vi "Init.vi"(8 "error in (no error)":errorcluster) -> (0 "error out":errorcluster, 3 "Message Queues out":T1)   [LabVIEW 2017, in "Server.lvlib"]
doc: "This VI creates all Message Queues and User Events, initializes the ErrorHandler and the Stop-Global Variable."
uses:
  Server.lvlib
  SubLibs/Message Queue/CommReferences.ctl
  SubLibs/Message Queue/MessageCluster.ctl
  SubLibs/Message Queue/EnqueueMessage(Single).vi
  SubLibs/Message Queue/Message Queue.lvlib
  SubLibs/ErrorLogger/ErrorLogger.lvlib
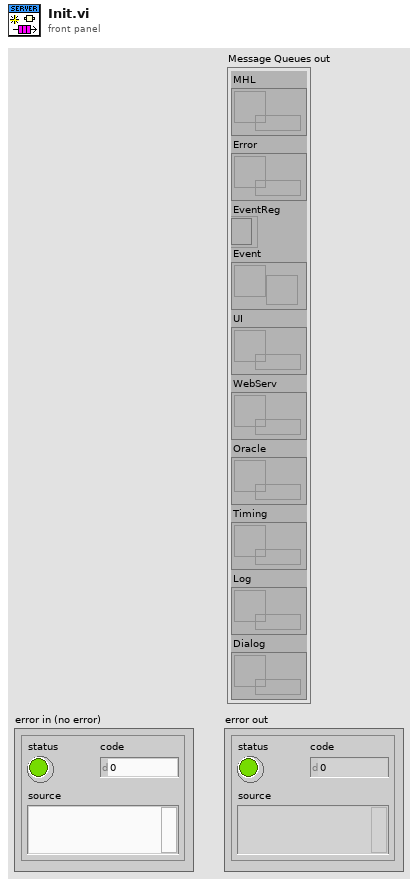
[diagram p1: front panel]
types:
  T1 = typedef "Server.lvlib/Message Queue.lvlib/CommReferences.ctl" = cluster{"MHL":refnum<queue>, "Error":refnum<queue>, "EventReg":refnum<event-registration>, "Event":refnum<user-event>, "UI":refnum<queue>, "WebServ":refnum<queue>, "Oracle":refnum<queue>, "Timing":refnum<queue>, "Log":refnum<queue>, "Dialog":refnum<queue>}
  T2 = typedef "Server.lvlib/ServerINI.ctl" = cluster{"ClientTimeout (s)":u32, "LogPath":path, "CriticalErrors":i32[], "OracleData":T3}
  T3 = typedef "Server.lvlib/Oracle.lvlib/OracleData.ctl" = cluster{"DBname":string, "User":string, "Password":string}
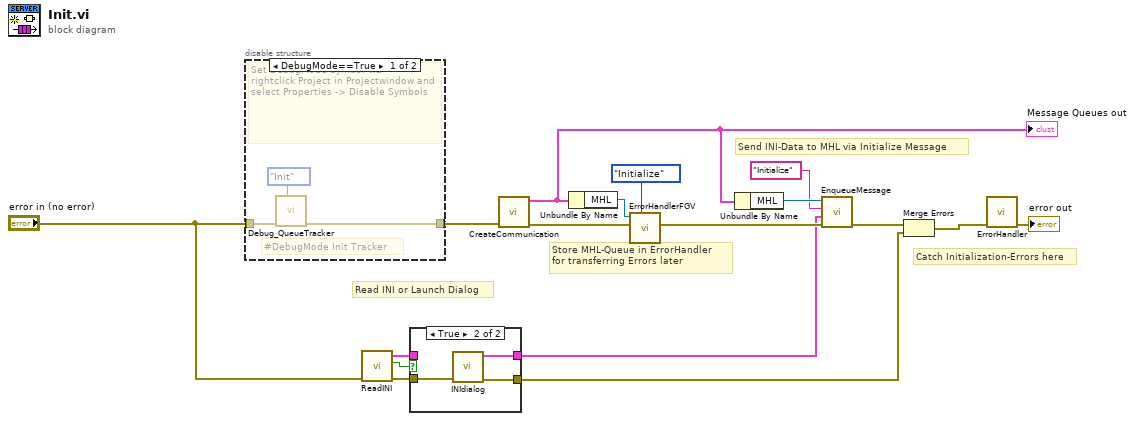
[diagram p0: block diagram]
diagram:
  # "Catch Initialization-Errors here"
  # "Send INI-Data to MHL via Initialize Message"
  # "Store MHL-Queue in ErrorHandler\nfor transferring Errors later"
  # "Read INI or Launch Dialog"
  n1 = disable-structure shown="DebugMode==True" {
    disable-tunnel: "error in (no error)" -> [w19 w21]
    disable-tunnel: [w18 w21] -> w10
    frame condition #0 {
      # "#DebugMode Init Tracker"
      # "Set DebugMode-Symbol via\nrightclick Project in Projectwindow and select Properties -> Disable Symbols"
      n2 = call "Debug_QueueTracker.vi"("Mode"=enum16{"Init", "Track", "DeInit"}."Init", "Error In"=w19) -> ("Error Out"=w18:errorcluster)  [unwired: 9 in]
    }
    frame condition #1 (active) {
      # "Don't track Queues if not in \nDebug-Mode.\nMode is settable in Project-file"
    }
  }
  n3 = call "ReadINI.vi"("error in (no error)"="error in (no error)") -> ("error out"=w12:errorcluster, "FileNotFound/Corrupted?"=w11:bool, "value"=w9:T2)  [unwired: 8 in]
  n4 = case shown="True" w11 {
    tunnel: w12 -> [w23 w26]
    tunnel: [w23 w25] -> w1
    tunnel: [w22 w24] -> w4
    tunnel: w9 -> [w22 _]
    frame False {
    }
    frame True {
      n5 = call "INIdialog.vi"("Error In"=w26) -> ("Error Out"=w25:errorcluster, "ServerINI"=w24:T2)  [unwired: 9 in]
    }
  }
  n6 = call "CreateCommunication.vi"("error in (no error)"=w10) -> ("error out"=w17:errorcluster, "Message Queues out"=w7:T1)  [unwired: 9 in]
  "Message Queues out" <- w7
  n7 = Unbundle By Name(w7) -> ("MHL"=w15:refnum<queue>)
  n8 = call "ErrorHandlerFGV.vi"("Command(CheckErrors)"=enum16{"Initialize", "CheckErrors"}."Initialize", "Error In"=w17, "MHL"=w15) -> ("Error Out"=w14:errorcluster)  [unwired: 8 in]
  n9 = Unbundle By Name(w7) -> ("MHL"=w6:refnum<queue>)
  n10 = call-poly "EnqueueMessage.vi"("error in (no error)"=w14, "Message Data"=w4, "Message"="Initialize", "Message Queue"=w6) -> ("error out"=w8:errorcluster)  [unwired: 6 in, 1 out]
  n11 = Merge Errors(w8, w1) -> (w2:errorcluster)
  n12 = call "ErrorHandler.vi"("error in (no error)"=w2) -> ("error out"=→"error out":errorcluster)  [unwired: 10 in]
